vi "addNode.vi"(0 "reference":refnum<class "CallNode.lvclass">, 1 "node":refnum<class "AbstractNode.lvclass">, 2 "point2D":T1 {"y" format="%.2f"; "x" format="%.2f"}, 5 "error in (no error)":errorcluster) -> (14 "reference out":refnum<class "CallNode.lvclass">, 15 "added":bool, 19 "error out":errorcluster)   [LabVIEW 2014, in "CallNode.lvclass"]
doc: "public boolean addNode(Node n, Point2D p)"
uses:
  <resource>/Framework/Providers/Open_GDS/UML/CallNode_class/CallNode.lvclass
  <resource>/Framework/Providers/Open_GDS/UML/AbstractNode_class/AbstractNode.lvclass
  <resource>/Framework/Providers/Open_GDS/UML/General/Point/Point Point2D.ctl
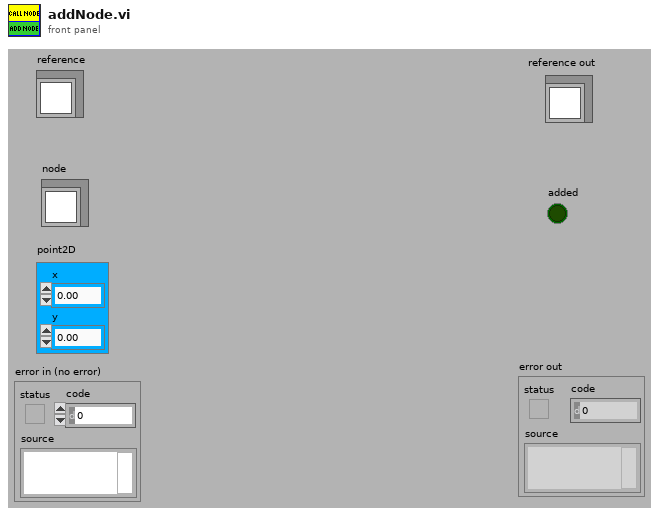
[diagram p1: front panel]
types:
  T1 = typedef "Point Point2D.ctl" = cluster{"x":dbl, "y":dbl}
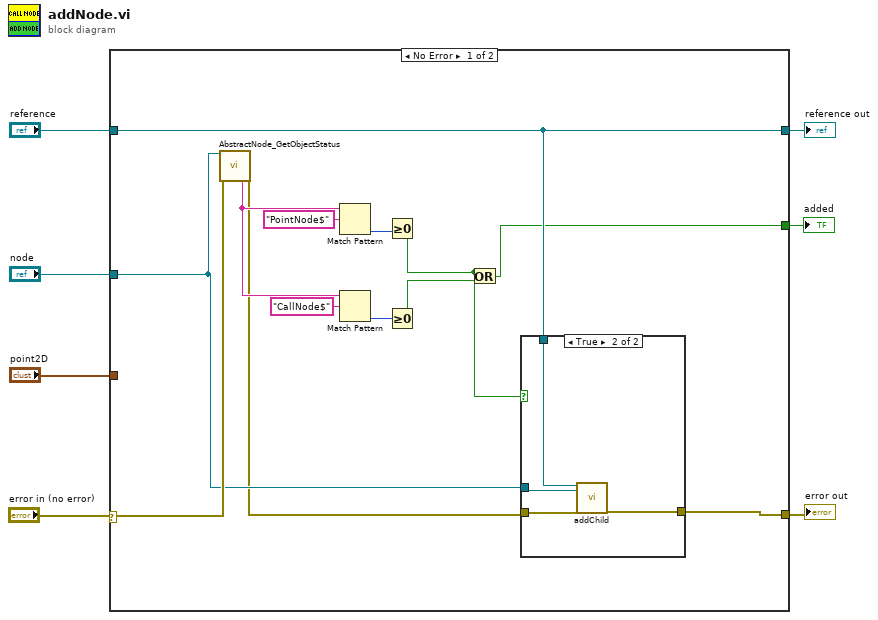
[diagram p0: block diagram]
diagram:
  n1 = case shown="No Error" "error in (no error)" {
    selector: "error in (no error)" -> [w18 w26]
    tunnel: "reference" -> [w20 w27]
    tunnel: [w19 w26] -> w6
    tunnel: [w20 w27] -> w5
    tunnel: "node" -> [w17 _]
    tunnel: "point2D" -> [_ _]
    tunnel: [w16 _] -> w1
    frame No Error {
      n2 = call <resource>:"AbstractNode_GetObjectStatus.vi"("reference in"=w17, "error in (no error)"=w18) -> ("Class name"=w12:string, "error out"=w9:errorcluster)  [unwired: 16 out]
      n3 = Match Pattern(string=w12, regular expression="PointNode$") -> (offset past match=w14:i32)  [unwired: 4 out]
      n4 = Match Pattern(string=w12, regular expression="CallNode$") -> (offset past match=w11:i32)  [unwired: 4 out]
      n5 = Greater Or Equal To 0?(x=w14) -> (x >= 0?=w8:bool)
      n6 = Greater Or Equal To 0?(x=w11) -> (x >= 0?=w10:bool)
      n7 = Or(x=w8, y=w10) -> (x .or. y?=w16:bool)
      n8 = case shown="True" w8 {
        tunnel: w9 -> [w21 w25]
        tunnel: [w21 w24] -> w19
        tunnel: w20 -> [_ w23]
        tunnel: w17 -> [_ w22]
        frame False {
        }
        frame True {
          n9 = call-dynamic "addChild.vi"("reference"=w23, "node"=w22, "error in (no error)"=w25) -> ("error out"=w24:errorcluster)  [unwired: 15 in, 1 out]
        }
      }
    }
    frame Error {
    }
  }
  "reference out" <- w5
  "error out" <- w6
  "added" <- w1
